vi "Set_BSA_voltage.vi"(0 "GPIB address":string, 2 "Desired Voltage":i16 min=0 max=1600, 3 "error in (no error)":errorcluster) -> (6 "Set Voltage":i32, 7 "error out":errorcluster)   [LabVIEW 2010]
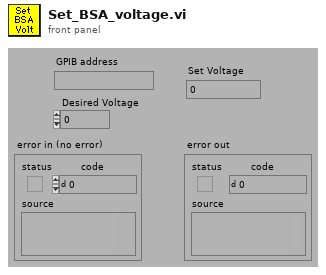
[diagram p1: front panel]
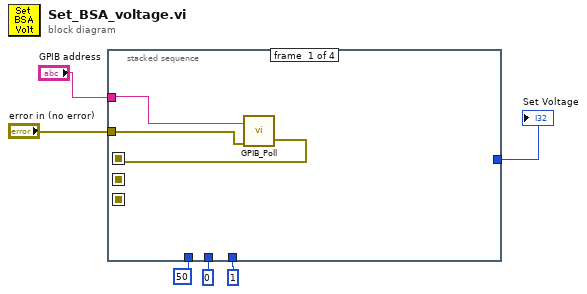
[diagram p0: block diagram]
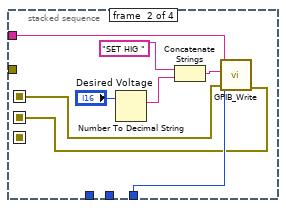
[diagram p2: hidden frame]
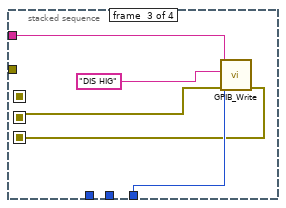
[diagram p3: hidden frame]
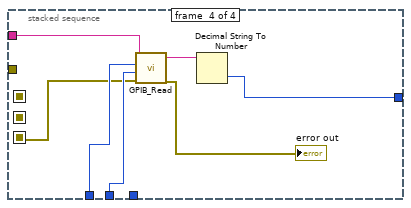
[diagram p4: hidden frame]
diagram:
  n1 = stacked-sequence {
    seq-local: [w7 _ _ _] -> [_ w11 _ _]
    seq-local: [_ w10 _ _] -> [_ _ w19 _]
    seq-local: [_ _ w18 _] -> [_ _ _ w24]
    tunnel: "GPIB address" -> [w9 w17 w22 w29]
    tunnel: 1 -> [_ w16 w21 _]
    tunnel: 0 -> [_ _ _ w28]
    tunnel: 50 -> [_ _ _ w27]
    tunnel: [_ _ _ w25] -> w2
    tunnel: "error in (no error)" -> [w8 _ _ _]
    frame #0 {
      n2 = call "GPIB_Poll.vi"("error in"=w8, "address string"=w9) -> ("error out"=w7:errorcluster)  [unwired: 1 out]
    }
    frame #1 {
      n3 = Number To Decimal String(number="Desired Voltage") -> (decimal integer string=w14:string)  [unwired: 1 out]
      n4 = Concatenate Strings("SET HIG ", w14) -> (w12:string)
      n5 = call "GPIB_Write.vi"("address string"=w17, "data In"=w12, "mode (0)"=w16, "error in"=w11) -> ("error out"=w10:errorcluster)  [unwired: 1 in, 1 out]
    }
    frame #2 {
      n6 = call "GPIB_Write.vi"("address string"=w22, "data In"="DIS HIG", "mode (0)"=w21, "error in"=w19) -> ("error out"=w18:errorcluster)  [unwired: 1 in, 1 out]
    }
    frame #3 {
      n7 = call "GPIB_Read.vi"("address string"=w29, "byte count"=w27, "mode (0)"=w28, "error in"=w24) -> ("data Out"=w26:string, "error out"=→"error out":errorcluster)  [unwired: 1 in, 1 out]
      n8 = Decimal String To Number(string=w26) -> (number=w25:i32)  [unwired: 3 out]
    }
  }
  "Set Voltage" <- w2
